vi "get_ellipsoid_params.vi"(8 "error in (no error)":errorcluster, 11 "RoiEllipsoid in":refnum<class "RoiEllipsoid.lvclass">=refnum) -> (0 "error out":errorcluster, 1 "b":dbl[unit], 2 "a":dbl[unit], 3 "RoiEllipsoid out":refnum<class "RoiEllipsoid.lvclass">, 4 "c":dbl[unit])   [LabVIEW 2010, in "RoiEllipsoid.lvclass"]
uses:
  RoiEllipsoid.lvclass
  common/classes/Box/Box/Box.lvclass
  common/classes/SpaceVector/SpaceVector/SpaceVector.lvclass
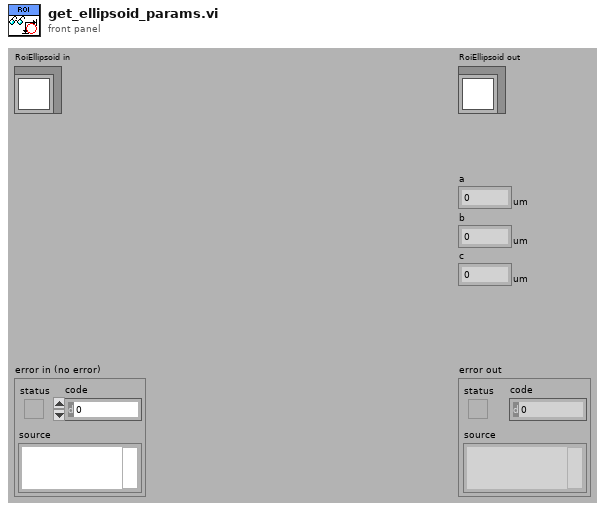
[diagram p1: front panel]
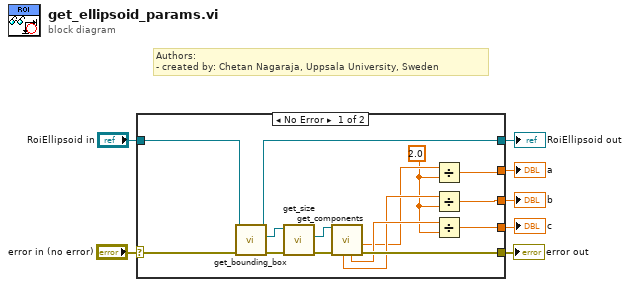
[diagram p0: block diagram]
diagram:
  # "Authors: \n- created by: Chetan Nagaraja, Uppsala University, Sweden"
  n1 = case shown="No Error" "error in (no error)" {
    selector: "error in (no error)" -> [w19 w24]
    tunnel: [w21 w24] -> w6
    tunnel: [w8 w23] -> w4
    tunnel: "RoiEllipsoid in" -> [w9 w23]
    tunnel: [w11 _] -> w3
    tunnel: [w12 _] -> w2
    tunnel: [w10 _] -> w1
    frame No Error {
      w13 = 2.0 ("y")
      n2 = call-dynamic "get_bounding_box.vi"("error in (no error)"=w19, "RoiGeneric in"=w9) -> ("error out"=w18:errorcluster, "Box.lvclass"=w17:refnum<class "Box.lvclass">, "RoiGeneric out"=w8:refnum<class "RoiEllipsoid.lvclass">)  [unwired: 7 in]
      n3 = call "get_size.vi"("error in (no error)"=w18, "Box in"=w17) -> ("error out"=w22:errorcluster, "size"=w20:refnum<class "SpaceVector.lvclass">)  [unwired: 7 in, 1 out]
      n4 = call "get_components.vi"("error in (no error)"=w22, "SpaceVector in"=w20) -> ("error out"=w21:errorcluster, "x"=w14:dbl[unit], "z"=w16:dbl[unit], "y"=w15:dbl[unit])  [unwired: 4 in, 2 out]
      n5 = Divide(x=w14, y=w13) -> (x/y=w11:dbl[unit])
      n6 = Divide(x=w15, y=w13) -> (x/y=w12:dbl[unit])
      n7 = Divide(x=w16, y=w13) -> (x/y=w10:dbl[unit])
    }
    frame Error {
    }
  }
  "error out" <- w6
  "RoiEllipsoid out" <- w4
  "a" <- w3
  "b" <- w2
  "c" <- w1
